vi "Rotate 90.vi"(6 "Rotate":T2, 8 "error in (no error)":errorcluster, 11 "Image Src":T1) -> (0 "error out":errorcluster, 3 "Image Dst Out":T1)   [LabVIEW 2015, in "Camera SubVIs.lvlib"]
uses:
  Camera SubVIs.lvlib
  Rotate.ctl
  <vilib>/vision/Image Controls.llb/IMAQ Image.ctl
  <vilib>/vision/NI_Vision_Development_Module.lvlib
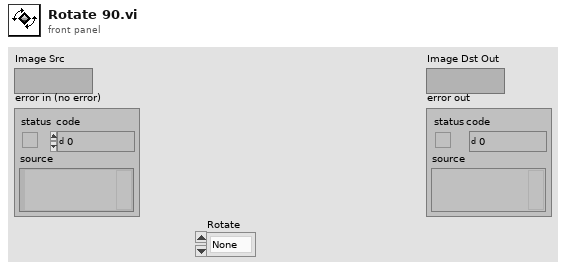
[diagram p1: front panel]
types:
  T1 = typedef "IMAQ Image.ctl" = refnum<image>
  T2 = typedef "Camera SubVIs.lvlib/Rotate.ctl" = enum16{"None", "CW", "CCW"}
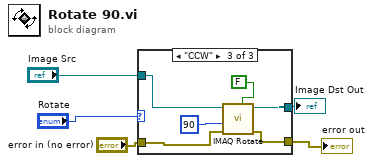
[diagram p0: block diagram]
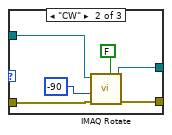
[diagram p3: hidden frame]
diagram:
  n1 = case shown="\"CCW\"" "Rotate" {
    tunnel: "Image Src" -> [w7 w12 w18]
    tunnel: [w7 w11 w17] -> w3
    tunnel: [w6 w10 w15] -> w2
    tunnel: "error in (no error)" -> [w6 w9 w16]
    frame "None", Default {
    }
    frame "CW" {
      n2 = call "IMAQ Rotate"("Maintain Size"=FALSE, "error in (no error)"=w9, "Angle (degrees)"=-90, "Image Src"=w12) -> ("error out"=w10:errorcluster, "Image Dst Out"=w11:T1)  [unwired: 6 in]
    }
    frame "CCW" {
      n3 = call "IMAQ Rotate"("Maintain Size"=FALSE, "error in (no error)"=w16, "Angle (degrees)"=90, "Image Src"=w18) -> ("error out"=w15:errorcluster, "Image Dst Out"=w17:T1)  [unwired: 6 in]
    }
  }
  "Image Dst Out" <- w3
  "error out" <- w2
